vi "Calculate read progress.vi"(4 "TDMS controls in":T1[][](array[typedef]), 5 "Playback Options":T2 {"chunks" format="%.0p"; "Samples per Write" format="%.3p"}) -> (1 "Read progress [%]":dbl[](array[numeric]))   [LabVIEW 2016]
uses:
  TypeDefs/Playback Options.ctl
  TypeDefs/TDMS read.ctl
panel:
  out "Error Out":errorcluster
  in  "Error In":errorcluster
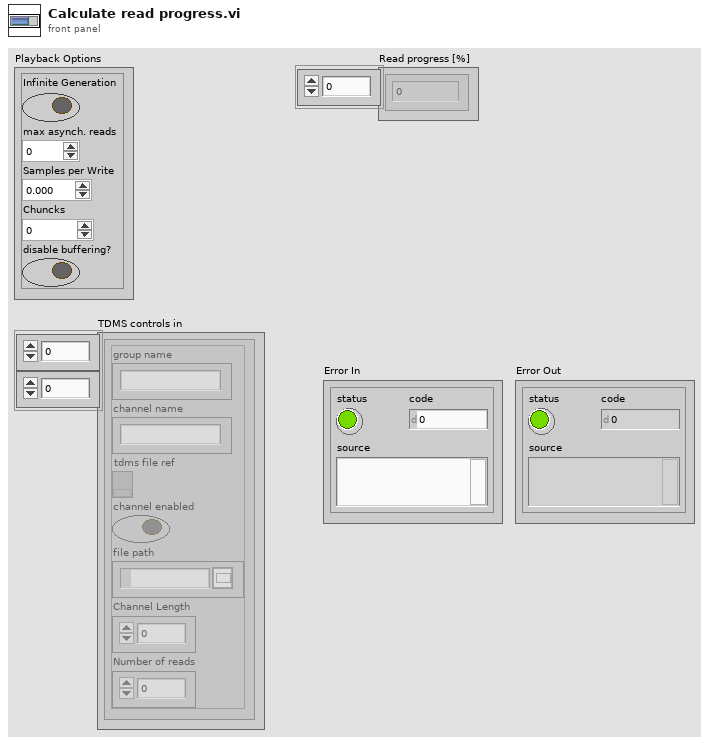
[diagram p1: front panel]
types:
  T1 = typedef "TDMS read.ctl" = cluster{"group name":string, "channel name":string, "tdms file ref":refnum<k34>, "channel enabled":bool, "file path":path, "Channel Length":i64, "Number of reads":i64}
  T2 = typedef "Playback Options.ctl" = cluster{"Infinite Generation":bool, "max asynch. reads":u32, "Samples per Write":u32, "chunks":u32, "disable buffering?":bool}
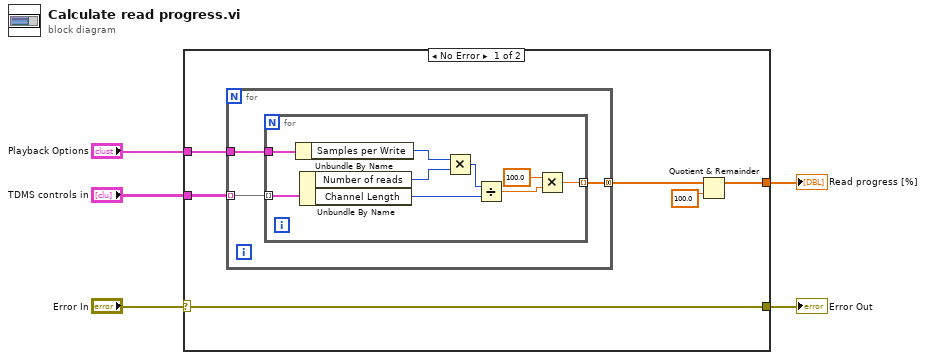
[diagram p0: block diagram]
diagram:
  n1 = case shown="No Error" "Error In" {
    selector: "Error In" -> [w9 w24]
    tunnel: [w6 _] -> w5
    tunnel: "Playback Options" -> [w11 _]
    tunnel: "TDMS controls in" -> [w10 _]
    tunnel: [w9 w24] -> w1
    frame No Error {
      n2 = for {
        tunnel: w10 -> [w14] mode=indexing
        tunnel: w11 -> [w13]
        tunnel: [w12] -> w7 mode=concatenating
        n3 = for {
          tunnel: w14 -> [w23] mode=indexing
          tunnel: w13 -> [w22]
          tunnel: [w16] -> w12 mode=indexing
          n4 = Unbundle By Name(w22) -> ("Samples per Write"=w19:u32)
          n5 = Unbundle By Name(w23) -> ("Number of reads"=w20:i64, "Channel Length"=w21:i64)
          n6 = Multiply(x=w19, y=w20) -> (x*y=w18:i64)
          n7 = Divide(x=w18, y=w21) -> (x/y=w17:dbl)
          n8 = Multiply(x=100.0, y=w17) -> (x*y=w16:dbl)
        }
      }
      n9 = Quotient & Remainder(x=w7, y=100.0) -> (x-y*floor(x/y)=w6:dbl[])  [unwired: 1 out]
    }
    frame Error {
    }
  }
  "Read progress [%]" <- w5
  "Error Out" <- w1
